vi "Storage Sample Out.vi"(8 "error in (no error)":errorcluster, 11 "Storage Line in":refnum<class "Storage Line.lvclass">=refnum) -> (0 "error out":errorcluster, 3 "Storage Line out":refnum<class "Storage Line.lvclass">)   [LabVIEW 2015]
uses:
  subs/Sample/Sample.lvclass
  Storage Line.lvclass
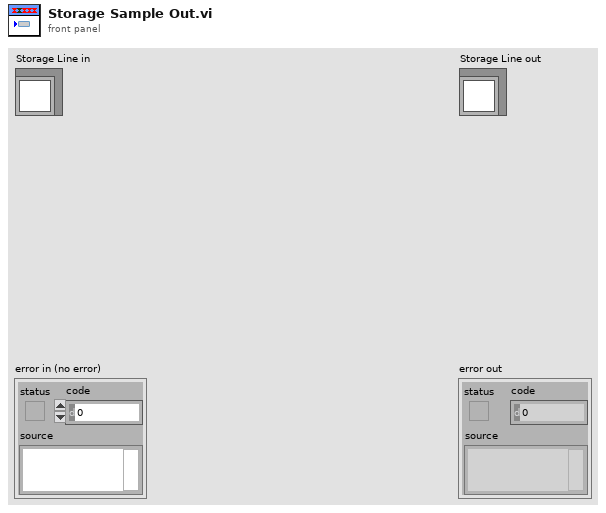
[diagram p1: front panel]
types:
  T1 = typedef "Sample Container SHV.ctl" = cluster{"Sample In":refnum<k21>, "Sample Name":refnum<k21>, "Ti Cathode":refnum<k21>, "Event":refnum<user-event>}
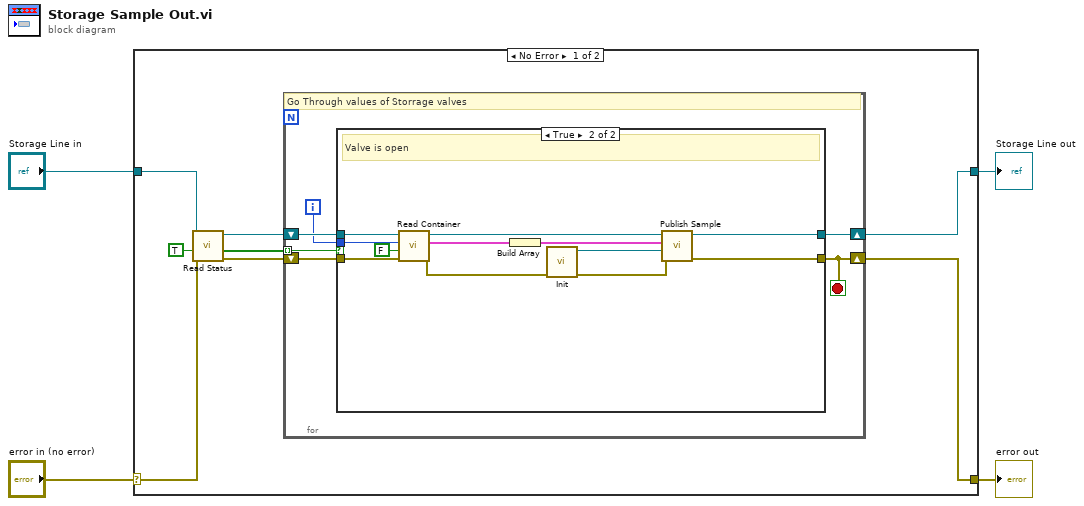
[diagram p0: block diagram]
diagram:
  n1 = case shown="No Error" "error in (no error)" {
    selector: "error in (no error)" -> [w7 w34]
    tunnel: [w6 w34] -> w4
    tunnel: [w5 w33] -> w2
    tunnel: "Storage Line in" -> [w10 w33]
    frame No Error {
      n2 = call "Read Status.vi"("error in (no error)"=w7, "Return Boolean Array? (F)"=TRUE, "Storage Line in"=w10) -> ("error out"=w8:errorcluster, "Boolean array"=w11:bool[], "Storage Line out"=w9:refnum<class "Storage Line.lvclass">)  [unwired: 5 in, 1 out]
      n3 = for {
        tunnel: w11 -> [w17] mode=indexing
        shift-right: [w16] -> w5
        shift-left: w9 -> [w18]
        shift-right: [w13] -> w6
        shift-left: w8 -> [w14]
        i -> [w15]
        stop <- w13 stop-if-true
        # "Go Through values of Storrage valves"
        n4 = case shown="True" w17 {
          tunnel: w18 -> [w20 w32]
          tunnel: [w20 w26] -> w16
          tunnel: w15 -> [_ w31]
          tunnel: w14 -> [w19 w30]
          tunnel: [w19 w25] -> w13
          frame False {
            # "Valve is closed"
          }
          frame True {
            # "Valve is open"
            n5 = call "Read Container.vi"("error in (no error)"=w30, "Read Sample (F)"=FALSE, "index"=w31, "Storage Line in"=w32) -> ("error out"=w23:errorcluster, "Tube SHV"=w27:T1, "Storage Line out"=w29:refnum<class "Storage Line.lvclass">)  [unwired: 4 in, 1 out]
            n6 = Build Array(w27) -> (w21:T1[])
            n7 = call "Init.vi"("error in (no error)"=w23) -> ("error out"=w28:errorcluster, "Sample out"=w22:refnum<class "Sample.lvclass">)  [unwired: 9 in]
            n8 = call-dynamic "Publish Sample.vi"("error in (no error)"=w28, "Sample"=w22, "Containers"=w21, "CO2 Actor in"=w29) -> ("error out"=w25:errorcluster, "CO2 Actor in 2"=w26:refnum<class "Storage Line.lvclass">)  [unwired: 6 in]
          }
        }
      }
    }
    frame Error {
    }
  }
  "error out" <- w4
  "Storage Line out" <- w2
